vi "Set Hostname Ctrl.vi"(8 "Error In":errorcluster, 11 "Hostname":string) -> (0 "Error Out":errorcluster)   [LabVIEW 2019, in "LMH-LINX.lvlib"]
uses:
  <vilib>/MakerHub/LINX/LMH-LINX.lvlib
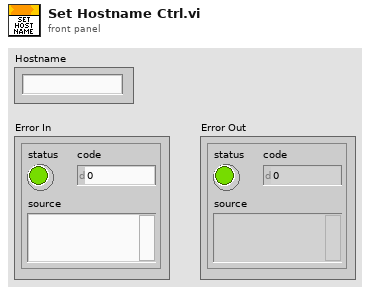
[diagram p1: front panel]
types:
  T1 = typedef "LMH-LINX.lvlib/Network Settings Ctrl Refs.ctl" = cluster{"Hostname":refnum<vi>, "IP address":refnum<vi>, "Subnet mask":refnum<vi>, "Default Gateway":refnum<vi>, "SSID":refnum<vi>, "Password":refnum<vi>, "NIC Status":refnum<vi>, "Network Interface":refnum<vi>, "DCHP":refnum<vi>}
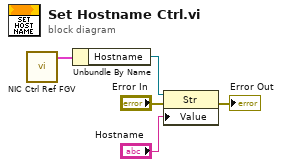
[diagram p0: block diagram]
diagram:
  n1 = call <vilib>:"NIC Ctrl Ref FGV.vi"() -> ("Network Settings Ctrl Refs"=w1:T1)  [unwired: 4 in]
  n2 = Unbundle By Name(w1) -> ("Hostname"=w2:refnum<vi>)
  n3 = property class="Str"(reference=w2, error in="Error In", "Value"="Hostname") -> (error out=→"Error Out":errorcluster)  [unwired: 1 out]
